vi "month_txt.vi"() -> ()   [LabVIEW 2017]
panel:
  in  "month_txt":dbl
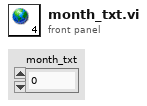
[diagram p1: front panel]
diagram:
